vi "Standalone REST (RT).vi"() -> ()   [LabVIEW 2023]
uses:
  Log/Log_Level.ctl
  API Message/API Message.lvclass
  Log/Log_Facilities.ctl
  Response/Standard Response Messages.ctl
  5ff5fe4d-644e-42b3-82e9-72adbb7d47a0.vi
  701e6035-b014-4147-aab3-b3ce1f9fae1e.vi
  5a67b58a-d501-4dc3-8558-0c804d545b7c.vi
  e8db4eca-cc96-4f6d-a0d1-e29095bc51eb.vi
  1441fe33-22a0-4e61-8bdf-aaa6b22bb0fa.vi
  c70d4357-6874-4551-bf72-0a3070db1cee.vi
  baea4f90-ed66-40c9-855f-b5689293d002.vi
  5ff5fe4d-644e-42b3-82e9-72adbb7d47a0.vi/bf0030c7-b76b-4182-9f9e-16cd2e366061.vi
  701e6035-b014-4147-aab3-b3ce1f9fae1e.vi/bf0030c7-b76b-4182-9f9e-16cd2e366061.vi
  5a67b58a-d501-4dc3-8558-0c804d545b7c.vi/bf0030c7-b76b-4182-9f9e-16cd2e366061.vi
  e8db4eca-cc96-4f6d-a0d1-e29095bc51eb.vi/bf0030c7-b76b-4182-9f9e-16cd2e366061.vi
  1441fe33-22a0-4e61-8bdf-aaa6b22bb0fa.vi/bf0030c7-b76b-4182-9f9e-16cd2e366061.vi
  c70d4357-6874-4551-bf72-0a3070db1cee.vi/bf0030c7-b76b-4182-9f9e-16cd2e366061.vi
  baea4f90-ed66-40c9-855f-b5689293d002.vi/bf0030c7-b76b-4182-9f9e-16cd2e366061.vi
  Request/Get Request.vi
  Response/Set Body.vi
  Response/Set Content Type.vi
  Response/Set Status Code.vi
  Response/Send.vi
  Request/Request.lvclass
  Response/Response.lvclass
  Log/Log.lvclass
  Server/Server.lvclass
panel:
  in  "Thing 2":string="Value 2"
  in  "Thing 1":string="Value 1"
  in  "stop":bool
  # "http://rt_computer:8081/thing/1"
  # "http://rt_computer:8081/thing/2"
  # "NOTE1: change \"rt_computer\" in the above links to the IP address of the RT\nSystem (cRIO/PXI/etc) - this should match the IP in the Project window."
  # "NOTE1: if you change the Listen port (on the block diagram) you need to\nchange the URL to match.  e.g. http://rt_computer:8080/thing/1 for port 8080"
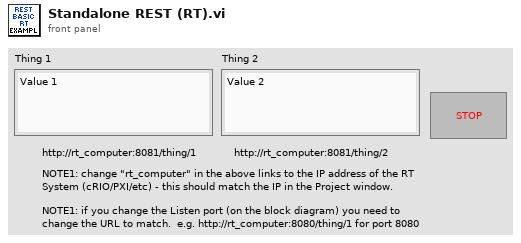
[diagram p1: front panel]
types:
  T1 = typedef "Log.lvclass/Log_Level.ctl" = enum16{"none", "info", "trace", "warn", "error", "fatal"}
  T2 = typedef "Log.lvclass/Log_Facilities.ctl" = string
  T3 = typedef "Request.ctl" = cluster{"Method":string, "URI":string, "Protocol":string, "Raw Path":string, "Query":string, "Fragment":string, "Raw Body":string, "Headers":variant, "Parameters":variant, "Body":variant, "Raw Header":string, "Path":string[]}
  T4 = typedef "Response.lvclass/Standard Response Messages.ctl" = u16
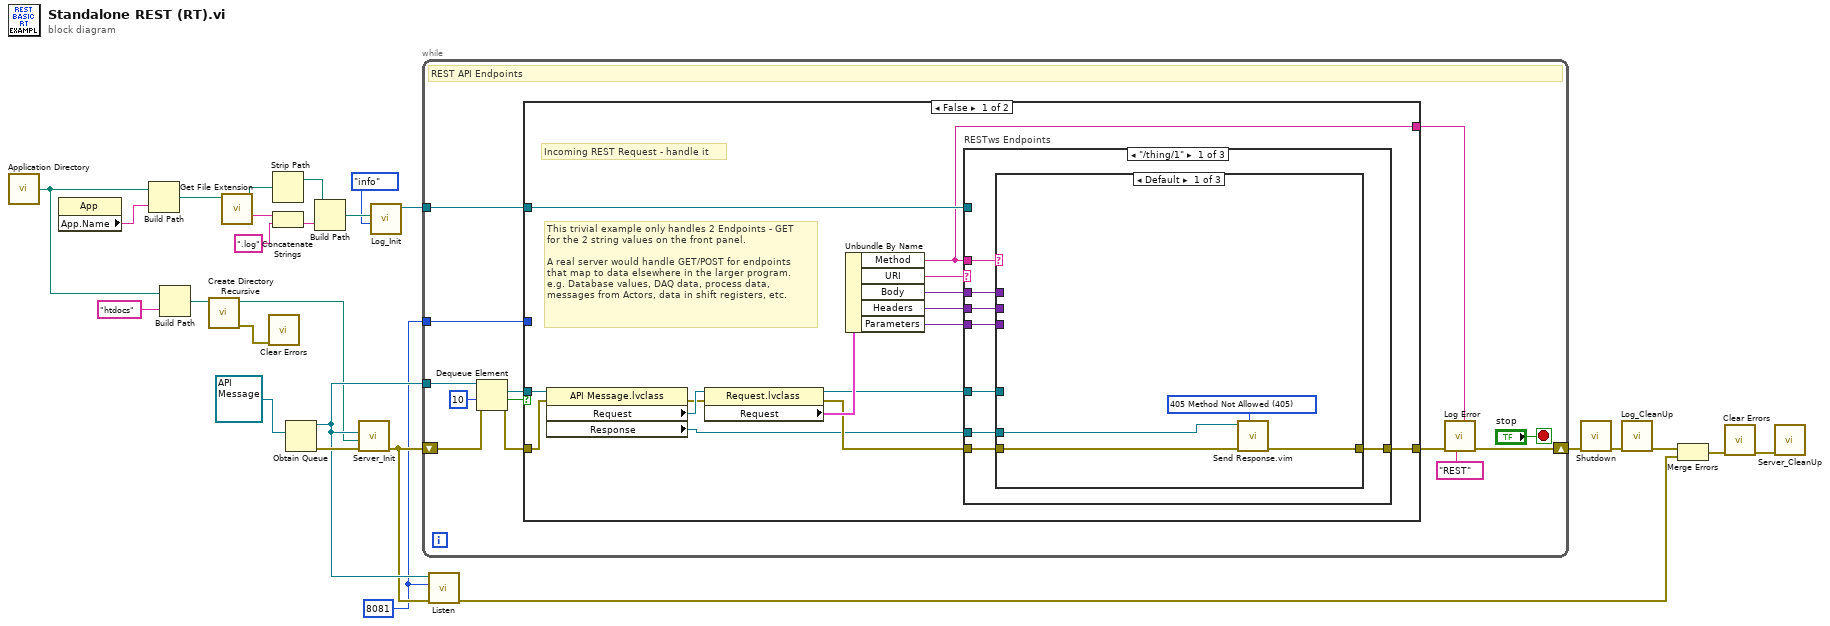
[diagram p0: block diagram]
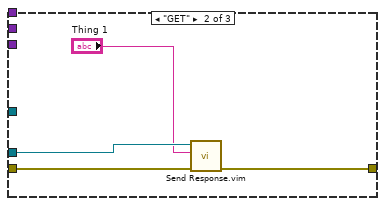
[diagram p2: hidden frame]
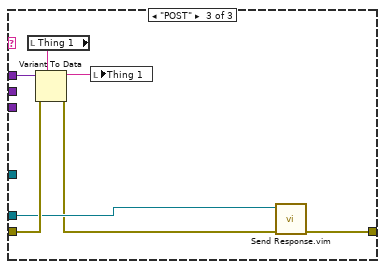
[diagram p3: hidden frame]
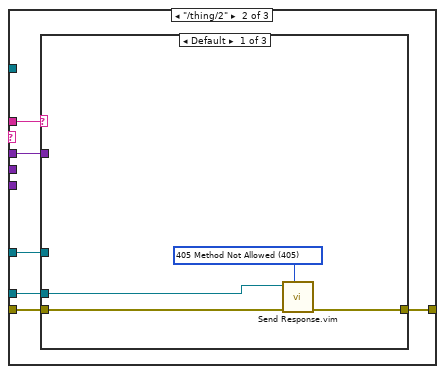
[diagram p4: hidden frame]
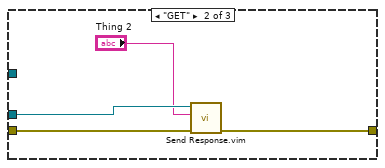
[diagram p5: hidden frame]
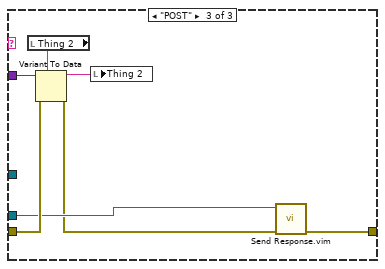
[diagram p6: hidden frame]
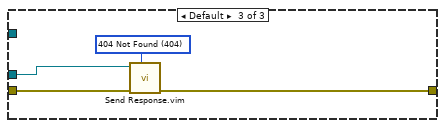
[diagram p7: hidden frame]
diagram:
  w4 = u16 8081 ("Listen Port (80)")
  n1 = call <vilib>:"Application Directory.vi"() -> ("Application Directory"=w17:path)
  n2 = property class="App"() -> ("App.Name"=w12:string)  [unwired: 2 in, 2 out]
  n3 = Build Path(base path=w17, name or relative path=w12) -> (appended path=w14:path)
  n4 = Build Path(base path=w17, name or relative path="htdocs" ("section")) -> (appended path=w3:path)
  n5 = call <vilib>:"Create Directory Recursive.vi"("directory"=w3) -> ("error out"=w1:errorcluster, "directory copy"=w2:path)  [unwired: 4 in, 1 out]
  n6 = call <vilib>:"Get File Extension.vi"("file"=w14) -> ("filename without extension"=w22:string, "dup file"=w21:path)  [unwired: 6 in, 3 out]
  n7 = call <vilib>:"Clear Errors.vi"("error in (no error)"=w1) -> ()  [unwired: 5 in, 2 out]
  n8 = Strip Path(path=w21) -> (stripped path=w20:path)  [unwired: 1 out]
  n9 = Concatenate Strings(w22, ".log" ("section")) -> (w25:string)
  n10 = Obtain Queue(element data type=refnum<class "API Message.lvclass"> refnum ("API Message.lvclass")) -> (queue out=w15:refnum<queue>, error out=w19:errorcluster)  [unwired: 4 in, 1 out]
  n11 = Build Path(base path=w20, name or relative path=w25) -> (appended path=w24:path)
  n12 = call "Server_Init.vi"("error in (no error)"=w19, "Static Data Folder"=w2, "API Queue"=w15) -> ("error out"=w13:errorcluster)  [unwired: 7 in, 1 out]
  n13 = call "Log_Init.vi"("Level"=Log_Level."info", "Log File"=w24) -> ("reference out"=w9:refnum<class "Log.lvclass">)  [unwired: 8 in, 1 out]
  n14 = while "Send to RT" {
    shift-right: [w30] -> w7
    shift-left: w13 -> [w34]
    tunnel: w15 -> [w39]
    tunnel: w9 -> [w32]
    tunnel: w4 -> [w27]
    stop <- "stop" stop-if-true
    # "REST API Endpoints"
    n15 = Dequeue Element(queue=w39, timeout in ms (-1)=10, error in (no error)=w34) -> (element=w36:refnum<class "API Message.lvclass">, timed out?=w38:bool, error out=w37:errorcluster)  [unwired: 1 out]
    n16 = case shown="False" w38 {
      tunnel: w37 -> [w53 w103]
      tunnel: [w47 w103] -> w31
      tunnel: w36 -> [w54 _]
      tunnel: w32 -> [w43 _]
      tunnel: [w42 _] -> w28
      tunnel: w27 -> [_ _]
      frame False {
        # "This trivial example only handles 2 Endpoints - GET\nfor the 2 string values on the front panel.\n\nA real server would handle GET/POST for endpoints\nthat map to data elsewhere in the larger program.\ne.g. Database values, DAQ data, process data, \nmessages from Actors, data in shift registers, etc."
        # "Incoming REST Request - handle it"
        n17 = property class="API Message.lvclass"(reference=w54, error in=w53) -> (error out=w51:errorcluster, "Request"=w52:refnum<class "Request.lvclass">, "Response"=w45:refnum<class "Response.lvclass">)  [unwired: 1 out]
        n18 = property class="Request.lvclass"(reference=w52, error in=w51) -> (reference out=w46:refnum<class "Request.lvclass">, error out=w48:errorcluster, "Request"=w50:T3)
        n19 = Unbundle By Name(w50) -> ("Method"=w42:string, "URI"=w49:string, "Body"=w44:variant, "Headers"=w41:variant, "Parameters"=w40:variant)
        n20 = case "RESTws Endpoints" shown="\"/thing/1\"" w49 {
          tunnel: w48 -> [w61 w82 w101]
          tunnel: [w62 w83 w102] -> w47
          tunnel: w42 -> [w58 w79 _]
          tunnel: w46 -> [w60 w81 _]
          tunnel: w45 -> [w59 w80 w100]
          tunnel: w44 -> [w57 w78 _]
          tunnel: w43 -> [_ _ _]
          tunnel: w41 -> [w56 _ _]
          tunnel: w40 -> [w55 _ _]
          frame "/thing/1" {
            n21 = case shown="Default" w58 {
              tunnel: [w64 w69 w71] -> w62
              tunnel: w61 -> [w66 w70 w76]
              tunnel: w60 -> [_ _ _]
              tunnel: w59 -> [w65 w68 w74]
              tunnel: w57 -> [_ _ w77]
              tunnel: w56 -> [_ _ _]
              tunnel: w55 -> [_ _ _]
              frame Default {
                w63 = T4 405 items=["200 OK"=200, "201 Created"=201, "202 Accepted"=202, "203 Non-Authoritative Information"=203, "204 No Content"=204, "205 Reset Content"=205, "206 Partial Content"=206, "207 Multi-Status (WebDAV)"=207, "208 Already Reported (WebDAV)"=208, "226 IM Used (HTTP Delta encoding)"=226, "300 Multiple Choices"=300, "301 Moved Permanently"=301, "302 Found"=302, "303 See Other"=303, "304 Not Modified"=304, "305 Use Proxy Deprecated"=305, "307 Temporary Redirect"=307, "308 Permanent Redirect"=308, "400 Bad Request"=400, "401 Unauthorized"=401, "402 Payment Required"=402, "403 Forbidden"=403, "404 Not Found"=404, "405 Method Not Allowed"=405, "406 Not Acceptable"=406, "407 Proxy Authentication Required"=407, "408 Request Timeout"=408, "409 Conflict"=409, "410 Gone"=410, "411 Length Required"=411, "412 Precondition Failed"=412, "413 Content Too Large"=413, "414 URI Too Long"=414, "415 Unsupported Media Type"=415, "416 Range Not Satisfiable"=416, "417 Expectation Failed"=417, "418 I'm a teapot"=418, "421 Misdirected Request"=421, "422 Unprocessable Content (WebDAV)"=422, "423 Locked (WebDAV)"=423, "424 Failed Dependency (WebDAV)"=424, "425 Too Early Experimental"=425, "426 Upgrade Required"=426, "428 Precondition Required"=428, "429 Too Many Requests"=429, "431 Request Header Fields Too Large"=431, "451 Unavailable For Legal Reasons"=451, "500 Internal Server Error"=500, "501 Not Implemented"=501, "502 Bad Gateway"=502, "503 Service Unavailable"=503, "504 Gateway Timeout"=504, "505 HTTP Version Not Supported"=505, "506 Variant Also Negotiates"=506, "507 Insufficient Storage (WebDAV)"=507, "508 Loop Detected (WebDAV)"=508, "510 Not Extended"=510, "511 Network Authentication Required"=511] ("Status Codes")
                n22 = call "Send Response.vim"("Status Code (200=OK)"=w63, "Error In"=w66, "Response"=w65) -> ("Error Out"=w64:errorcluster)  [unwired: 8 in]
              }
              frame "GET" {
                n23 = call "Send Response.vim"("Error In"=w70, "Body (\"\")"="Thing 1", "Response"=w68) -> ("Error Out"=w69:errorcluster)  [unwired: 8 in]
              }
              frame "POST" {
                n24 = local read "Thing 1"() -> (w72:string)
                n25 = Variant To Data(error in=w76, type=w72, Variant=w77) -> (data=w75:string, error out=w73:errorcluster)
                n26 = local write "Thing 1"(w75) -> ()
                n27 = call "Send Response.vim"("Error In"=w73, "Response"=w74) -> ("Error Out"=w71:errorcluster)  [unwired: 9 in]
              }
            }
          }
          frame "/thing/2" {
            n28 = case shown="Default" w79 {
              tunnel: [w85 w90 w92] -> w83
              tunnel: w82 -> [w87 w91 w97]
              tunnel: w81 -> [_ _ _]
              tunnel: w80 -> [w86 w89 w95]
              tunnel: w78 -> [_ _ w98]
              frame Default {
                w84 = T4 405 items=["200 OK"=200, "201 Created"=201, "202 Accepted"=202, "203 Non-Authoritative Information"=203, "204 No Content"=204, "205 Reset Content"=205, "206 Partial Content"=206, "207 Multi-Status (WebDAV)"=207, "208 Already Reported (WebDAV)"=208, "226 IM Used (HTTP Delta encoding)"=226, "300 Multiple Choices"=300, "301 Moved Permanently"=301, "302 Found"=302, "303 See Other"=303, "304 Not Modified"=304, "305 Use Proxy Deprecated"=305, "307 Temporary Redirect"=307, "308 Permanent Redirect"=308, "400 Bad Request"=400, "401 Unauthorized"=401, "402 Payment Required"=402, "403 Forbidden"=403, "404 Not Found"=404, "405 Method Not Allowed"=405, "406 Not Acceptable"=406, "407 Proxy Authentication Required"=407, "408 Request Timeout"=408, "409 Conflict"=409, "410 Gone"=410, "411 Length Required"=411, "412 Precondition Failed"=412, "413 Content Too Large"=413, "414 URI Too Long"=414, "415 Unsupported Media Type"=415, "416 Range Not Satisfiable"=416, "417 Expectation Failed"=417, "418 I'm a teapot"=418, "421 Misdirected Request"=421, "422 Unprocessable Content (WebDAV)"=422, "423 Locked (WebDAV)"=423, "424 Failed Dependency (WebDAV)"=424, "425 Too Early Experimental"=425, "426 Upgrade Required"=426, "428 Precondition Required"=428, "429 Too Many Requests"=429, "431 Request Header Fields Too Large"=431, "451 Unavailable For Legal Reasons"=451, "500 Internal Server Error"=500, "501 Not Implemented"=501, "502 Bad Gateway"=502, "503 Service Unavailable"=503, "504 Gateway Timeout"=504, "505 HTTP Version Not Supported"=505, "506 Variant Also Negotiates"=506, "507 Insufficient Storage (WebDAV)"=507, "508 Loop Detected (WebDAV)"=508, "510 Not Extended"=510, "511 Network Authentication Required"=511] ("Status Codes")
                n29 = call "Send Response.vim"("Status Code (200=OK)"=w84, "Error In"=w87, "Response"=w86) -> ("Error Out"=w85:errorcluster)  [unwired: 8 in]
              }
              frame "GET" {
                n30 = call "Send Response.vim"("Error In"=w91, "Body (\"\")"="Thing 2", "Response"=w89) -> ("Error Out"=w90:errorcluster)  [unwired: 8 in]
              }
              frame "POST" {
                n31 = local read "Thing 2"() -> (w93:string)
                n32 = Variant To Data(error in=w97, type=w93, Variant=w98) -> (data=w96:string, error out=w94:errorcluster)
                n33 = local write "Thing 2"(w96) -> ()
                n34 = call "Send Response.vim"("Error In"=w94, "Response"=w95) -> ("Error Out"=w92:errorcluster)  [unwired: 9 in]
              }
            }
          }
          frame Default {
            w99 = T4 404 items=["200 OK"=200, "201 Created"=201, "202 Accepted"=202, "203 Non-Authoritative Information"=203, "204 No Content"=204, "205 Reset Content"=205, "206 Partial Content"=206, "207 Multi-Status (WebDAV)"=207, "208 Already Reported (WebDAV)"=208, "226 IM Used (HTTP Delta encoding)"=226, "300 Multiple Choices"=300, "301 Moved Permanently"=301, "302 Found"=302, "303 See Other"=303, "304 Not Modified"=304, "305 Use Proxy Deprecated"=305, "307 Temporary Redirect"=307, "308 Permanent Redirect"=308, "400 Bad Request"=400, "401 Unauthorized"=401, "402 Payment Required"=402, "403 Forbidden"=403, "404 Not Found"=404, "405 Method Not Allowed"=405, "406 Not Acceptable"=406, "407 Proxy Authentication Required"=407, "408 Request Timeout"=408, "409 Conflict"=409, "410 Gone"=410, "411 Length Required"=411, "412 Precondition Failed"=412, "413 Content Too Large"=413, "414 URI Too Long"=414, "415 Unsupported Media Type"=415, "416 Range Not Satisfiable"=416, "417 Expectation Failed"=417, "418 I'm a teapot"=418, "421 Misdirected Request"=421, "422 Unprocessable Content (WebDAV)"=422, "423 Locked (WebDAV)"=423, "424 Failed Dependency (WebDAV)"=424, "425 Too Early Experimental"=425, "426 Upgrade Required"=426, "428 Precondition Required"=428, "429 Too Many Requests"=429, "431 Request Header Fields Too Large"=431, "451 Unavailable For Legal Reasons"=451, "500 Internal Server Error"=500, "501 Not Implemented"=501, "502 Bad Gateway"=502, "503 Service Unavailable"=503, "504 Gateway Timeout"=504, "505 HTTP Version Not Supported"=505, "506 Variant Also Negotiates"=506, "507 Insufficient Storage (WebDAV)"=507, "508 Loop Detected (WebDAV)"=508, "510 Not Extended"=510, "511 Network Authentication Required"=511] ("Status Codes")
            n35 = call "Send Response.vim"("Status Code (200=OK)"=w99, "Error In"=w101, "Response"=w100) -> ("Error Out"=w102:errorcluster)  [unwired: 8 in]
          }
        }
      }
      frame True {
        # "No REST Message"
      }
    }
    n36 = call "Log Error.vi"("Context"=w28, "Facility (default)"=T2 "REST", "error in (no error)"=w31) -> ("error out"=w30:errorcluster)  [unwired: 8 in]
  }
  n37 = call "Listen.vi"("error in (no error)"=w13, "Listen Port (80)"=w4, "API Queue"=w15) -> ("error out"=w10:errorcluster)  [unwired: 8 in]
  n38 = call "Shutdown.vi"("error in (no error)"=w7) -> ("error out"=w6:errorcluster)  [unwired: 10 in]
  n39 = call "Log_CleanUp.vi"("error in (no error)"=w6) -> ("error out"=w8:errorcluster)  [unwired: 10 in]
  n40 = Merge Errors(w8, w10) -> (w11:errorcluster)
  n41 = call <vilib>:"Clear Errors.vi"("error in (no error)"=w11) -> ("error out"=w5:errorcluster)  [unwired: 5 in, 1 out]
  n42 = call "Server_CleanUp.vi"("error in (no error)"=w5) -> ()  [unwired: 10 in, 1 out]
